vi "top_loop.vi"(0 "Input parameters":T4={"Measurement type"=enum."Debug", "Sensor type"=enum."HPK_8in_256", "Identifier"="test.txt", "Open after execution?"=FALSE, "Plot after execution?"=FALSE, "Display channel"=0, "Voltage Delay (s)"=0.5, "Switch Delay (s)"=0.01, "VISA resource name source"="", "VISA resource name DMM"="", "VISA resource name LCR"="", "Compliance  Level (A)"=10.0, "Voltage Limit (V)"=1000.0, "Data storage location"="", "Scan voltages"="", "Use source as DMM?"=FALSE, "LCR signal frequenzy (Hz)"=10.0, "DMM device"=enum."Keithley2001", "Sampling number"=1, "Use env. sensors on"=enum."Sensirion sht1x/7x", "Switchboard Handle"=0, "Use Switchboard"=FALSE, "LCR signal voltage (V)"=10000.0, "Repeat"=1, "Scan voltages IV"="", "Scan voltages CV"="", "Hex pad numbers?"=FALSE, "Set measurement type"=enum."Debug", "Custom pad scan"="", "IV voltage Delay (s)"=0.5, "CV voltage Delay (s)"=0.5, "Needle measurement?"=FALSE, "Comments"="test.txt", "LCR signal frequenzy (kHz)"=10.0, "Compliance  Level (uA)"=10.0, "Open Correction Array"=array2304x3[6912 elements], "Current set voltage"=0.0, "Last set voltage"=0.0, "Current channel"=0, "Last OpenCorrection index"=-1, "Total curr/vltg every x steps"=10, "Current channel iteration"=0, "No CV corrections"=FALSE, "Mapfile"="", "Corrfile"="", "IV voltage file"=path "", "CV voltage file"=path "", "IV Switch Delay (s)"=0.01, "CV Switch Delay (s)"=0.01, "Invert polarity"=FALSE, "Set debug dirs"=FALSE, "Is n on p"=FALSE} {"CV Switch Delay (s)" format="%#_13g"; "IV Switch Delay (s)" format="%#_13g"; "Last set voltage" format="%#_13g"; "Current set voltage" format="%#_13g"; "CV voltage Delay (s)" format="%#_13g"; "IV voltage Delay (s)" format="%#_13g"; "Voltage Limit (V)" format="%#_13g"; "Voltage Delay (s)" format="%#_13g"; "Switch Delay (s)" format="%#_13g"}, 5 "Dynamic data":T3, 7 "Front_panel_refs":T1, 11 "error in (no error)":errorcluster, 12 "Environmental data":T2) -> (4 "Input parameters out":T4={"Measurement type"=enum."Debug", "Sensor type"=enum."HPK_8in_256", "Identifier"="test.txt", "Open after execution?"=FALSE, "Plot after execution?"=FALSE, "Display channel"=0, "Voltage Delay (s)"=0.5, "Switch Delay (s)"=0.01, "VISA resource name source"="", "VISA resource name DMM"="", "VISA resource name LCR"="", "Compliance  Level (A)"=10.0, "Voltage Limit (V)"=1000.0, "Data storage location"="", "Scan voltages"="", "Use source as DMM?"=FALSE, "LCR signal frequenzy (Hz)"=10.0, "DMM device"=enum."Keithley2001", "Sampling number"=1, "Use env. sensors on"=enum."Sensirion sht1x/7x", "Switchboard Handle"=0, "Use Switchboard"=FALSE, "LCR signal voltage (V)"=10000.0, "Repeat"=1, "Scan voltages IV"="", "Scan voltages CV"="", "Hex pad numbers?"=FALSE, "Set measurement type"=enum."Debug", "Custom pad scan"="", "IV voltage Delay (s)"=0.5, "CV voltage Delay (s)"=0.5, "Needle measurement?"=FALSE, "Comments"="test.txt", "LCR signal frequenzy (kHz)"=10.0, "Compliance  Level (uA)"=10.0, "Open Correction Array"=array2304x3[6912 elements], "Current set voltage"=0.0, "Last set voltage"=0.0, "Current channel"=0, "Last OpenCorrection index"=-1, "Total curr/vltg every x steps"=10, "Current channel iteration"=0, "No CV corrections"=FALSE, "Mapfile"="", "Corrfile"="", "IV voltage file"=path "", "CV voltage file"=path "", "IV Switch Delay (s)"=0.01, "CV Switch Delay (s)"=0.01, "Invert polarity"=FALSE, "Set debug dirs"=FALSE, "Is n on p"=FALSE} {"CV Switch Delay (s)" format="%#_13g"; "IV Switch Delay (s)" format="%#_13g"; "Last set voltage" format="%#_13g"; "Current set voltage" format="%#_13g"; "CV voltage Delay (s)" format="%#_13g"; "IV voltage Delay (s)" format="%#_13g"; "Voltage Limit (V)" format="%#_13g"; "Voltage Delay (s)" format="%#_13g"; "Switch Delay (s)" format="%#_13g"}, 6 "Dynamic data out":T3, 8 "Front_panel_refs out":T1, 15 "error out":errorcluster)   [LabVIEW 2016]
doc: "The main loop function of the HexDAQ."
uses:
  input_params.ctl
  data_dynamic.ctl
  <extravilib>/ChannelInstances/Tag-t'Env_data.ctl'/))Channel.ctl
  data_env.ctl
  refs_front_panel.ctl
  data_live.ctl
  <extravilib>/ChannelInstances/Tag-t'Env_data.ctl'/Read With Abort.vi
  <extravilib>/ChannelInstances/Tag-t'Env_data.ctl'/Endpoint.vi
  <extravilib>/ChannelInstances/Tag-t'Env_data.ctl'.lvlib
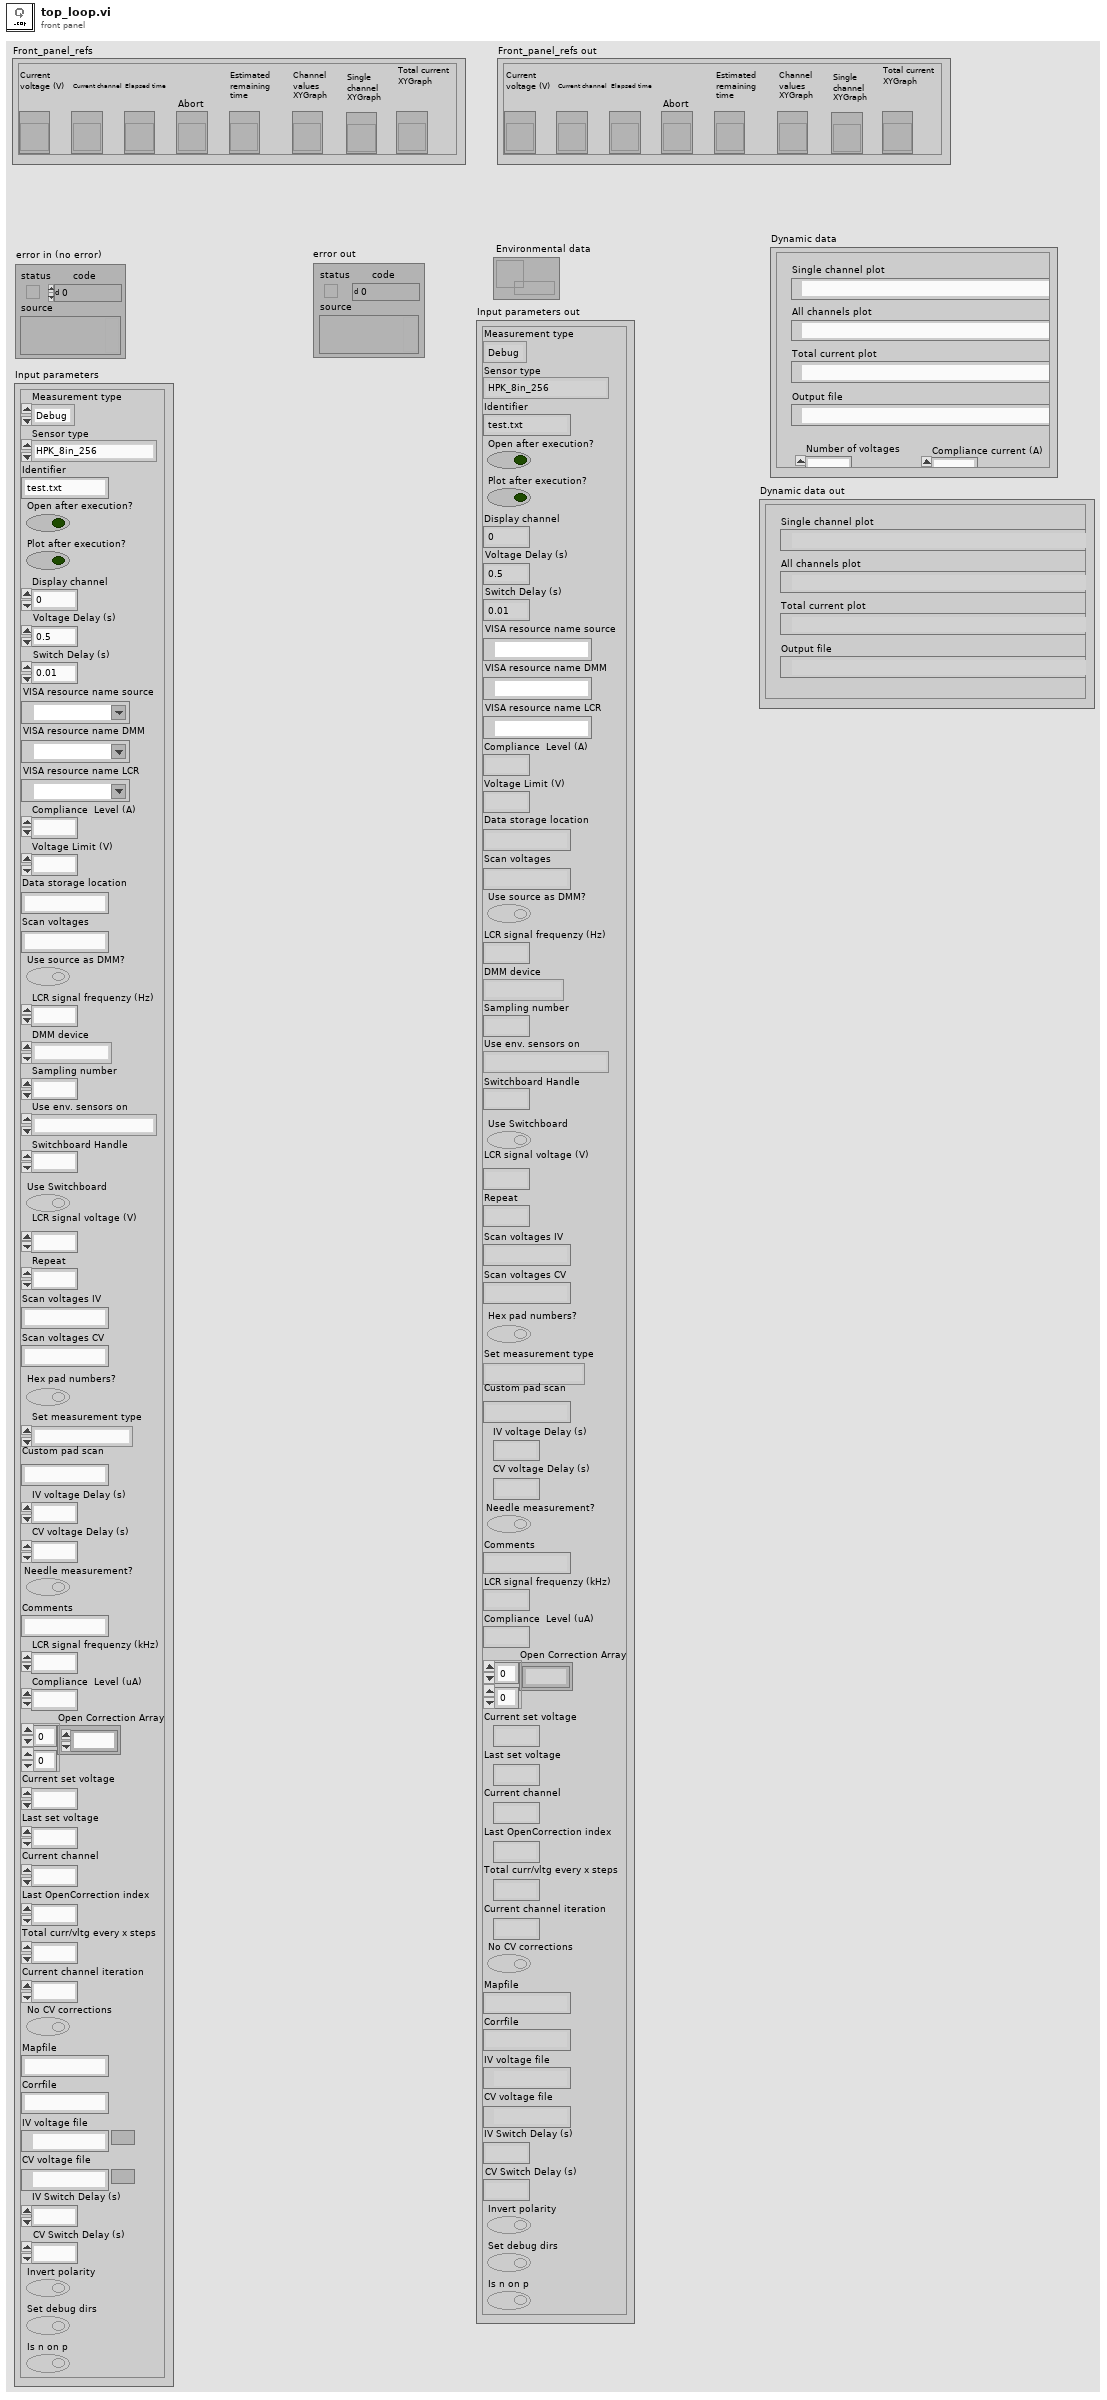
[diagram p1: front panel]
types:
  T1 = typedef "refs_front_panel.ctl" = cluster{"Current voltage (V)":refnum<vi>, "Elapsed time":refnum<vi>, "Current channel":refnum<vi>, "Abort":refnum<vi>, "Estimated remaining time":refnum<vi>, "Channel values XYGraph":refnum<vi>, "Single channel XYGraph":refnum<vi>, "Total current XYGraph":refnum<vi>}
  T2 = typedef "Tag-t'Env_data.ctl'.lvlib/))Channel.ctl" = refnum<queue>
  T3 = typedef "data_dynamic.ctl" = cluster{"Output file":path, "Y-label text":string, "Current set voltage":dbl, "Set voltage column":dbl[], "Pad number column":dbl[], "Data  column":dbl[], "Number of voltages":i32, "Compliance current (A)":dbl, "Geofile":string, "Peak voltage":dbl, "Hex PDF file":string, "Voltage array":dbl[], "Total current column":dbl[], "Timestamp column":dbl[], "Data name":string, "Data unit":string, "2nd data column":dbl[], "2nd data name":string, "2nd data unit":string, "3rd data column":dbl[], "4th data column":dbl[], "3rd data name":string, "3rd data unit":string, "4th data name":string, "4th data unit":string, "Actual voltage column":dbl[], "2nd Y-label text":string, "Single channel plot":path, "Temperature column":dbl[], "Humidity column":dbl[], "Channel switch array":i32[], "1st single plot name":string, "2nd single plot name":string, "All channels plot":path, "HexPlot command":string, "Custom channel array":i32[], "Data  error column":dbl[], "2nd data  error column":dbl[], "3rd data error column":dbl[], "4th data  error column":dbl[], "Total current plot":path, "5th data column":dbl[], "5th data  error column":dbl[], "6th data column":dbl[], "6th data  error column":dbl[], "5th data name":string, "5th data unit":string, "6th data name":string, "6th data unit":string, "HexPlot matrix command":string}
  T4 = typedef "input_params.ctl" = cluster{"Measurement type":enum16{"IV", "CV", "Debug", "Test_contact"}, "Sensor type":enum16{"HPK_6in_135", "HPK_8in_256", "IFX_8in_256", "Diode", "HPK_6in_256", "Full matrix"}, "Identifier":string, "Open after execution?":bool, "Plot after execution?":bool, "Display channel":i32, "Voltage Delay (s)":dbl, "Switch Delay (s)":dbl, "VISA resource name source":refnum<visa-resource-name>, "VISA resource name DMM":refnum<visa-resource-name>, "VISA resource name LCR":refnum<visa-resource-name>, "Compliance  Level (A)":dbl, "Voltage Limit (V)":dbl, "Data storage location":string, "Scan voltages":string, "Use source as DMM?":bool, "LCR signal frequenzy (Hz)":dbl, "DMM device":enum16{"Keithley2001", "Keithley2450", "Keithley2410", "Keithley6487"}, "Sampling number":i32, "Use env. sensors on":enum16{"Sensirion sht1x/7x", "Switch Matrix", "Probecard"}, "Switchboard Handle":u32, "Use Switchboard":bool, "LCR signal voltage (V)":dbl, "Repeat":i32, "Scan voltages IV":string, "Scan voltages CV":string, "Hex pad numbers?":bool, "Set measurement type":enum16{"IV", "CV", "Debug", "Test_contact", "IV+CV"}, "Custom pad scan":string, "IV voltage Delay (s)":dbl, "CV voltage Delay (s)":dbl, "Needle measurement?":bool, "Comments":string, "LCR signal frequenzy (kHz)":dbl, "Compliance  Level (uA)":dbl, "Open Correction Array":dbl[][], "Current set voltage":dbl, "Last set voltage":dbl, "Current channel":i32, "Last OpenCorrection index":i32, "Total curr/vltg every x steps":i32, "Current channel iteration":i32, "No CV corrections":bool, "Mapfile":string, "Corrfile":string, "IV voltage file":path, "CV voltage file":path, "IV Switch Delay (s)":dbl, "CV Switch Delay (s)":dbl, "Invert polarity":bool, "Set debug dirs":bool, "Is n on p":bool}
  T5 = typedef "data_live.ctl" = cluster{"Actual voltage":dbl, "Total current":dbl, "Data":dbl, "Data error":dbl, "2nd data":dbl, "2nd data error":dbl, "3rd data":dbl, "3rd data error":dbl, "4th data":dbl, "4th data error":dbl, "6th data error":dbl, "6th data":dbl, "5th data error":dbl, "5th data":dbl}
  T6 = enum16{"Sensirion sht1x/7x", "Switch Matrix", "Probecard"}
  T7 = typedef "data_env.ctl" = cluster{"Temp. Sensirion":dbl, "Hum. Sensirion":dbl, "Temp. Switch Matrix":dbl, "Hum. Switch Matrix":dbl, "Temp. Probecard":dbl, "Hum. Probecard":dbl}
  T8 = cluster{"XY Graph out":cluster{"Array":dbl[], "Array":dbl[]}[], "XY Graph out":cluster{"Array":dbl[], "Array":dbl[]}[]}
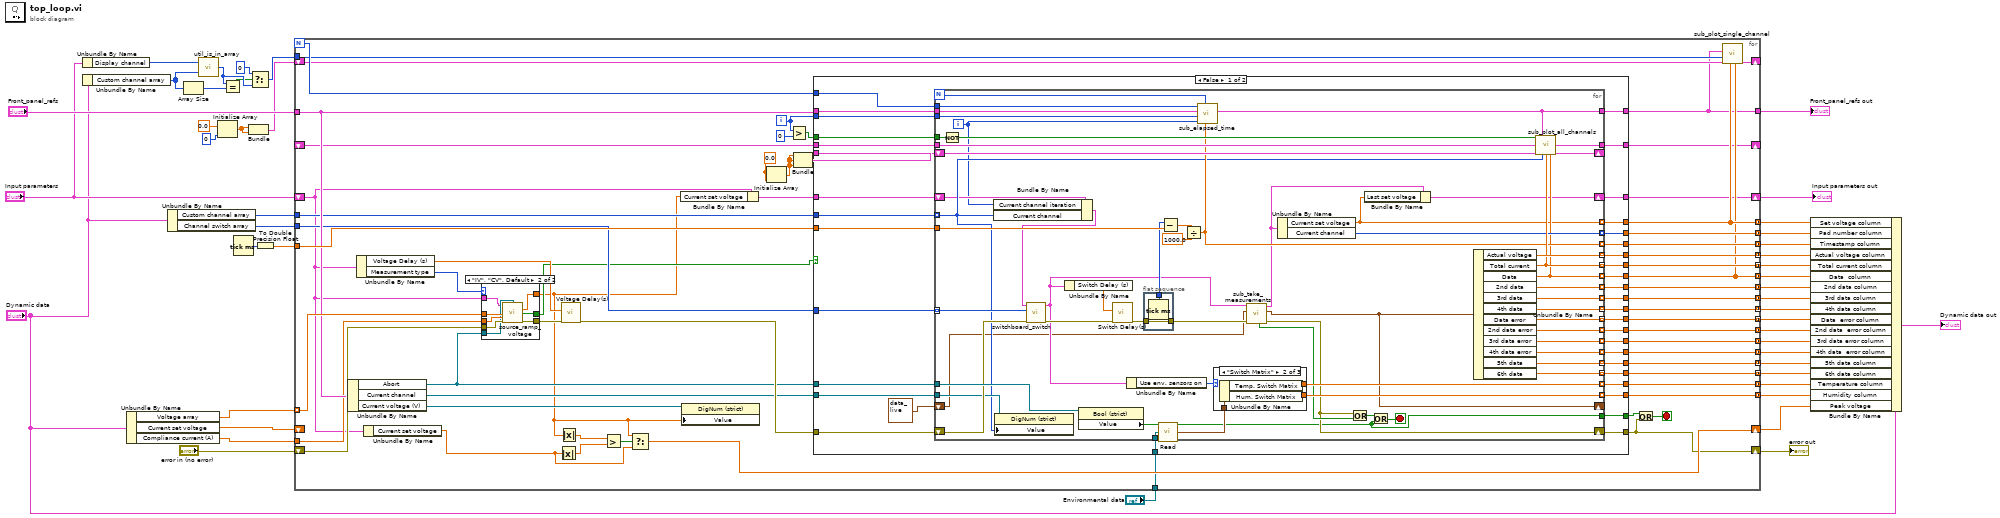
[diagram p0: block diagram]
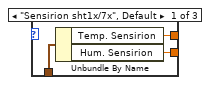
[diagram p2: hidden frame]
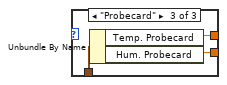
[diagram p3: hidden frame]
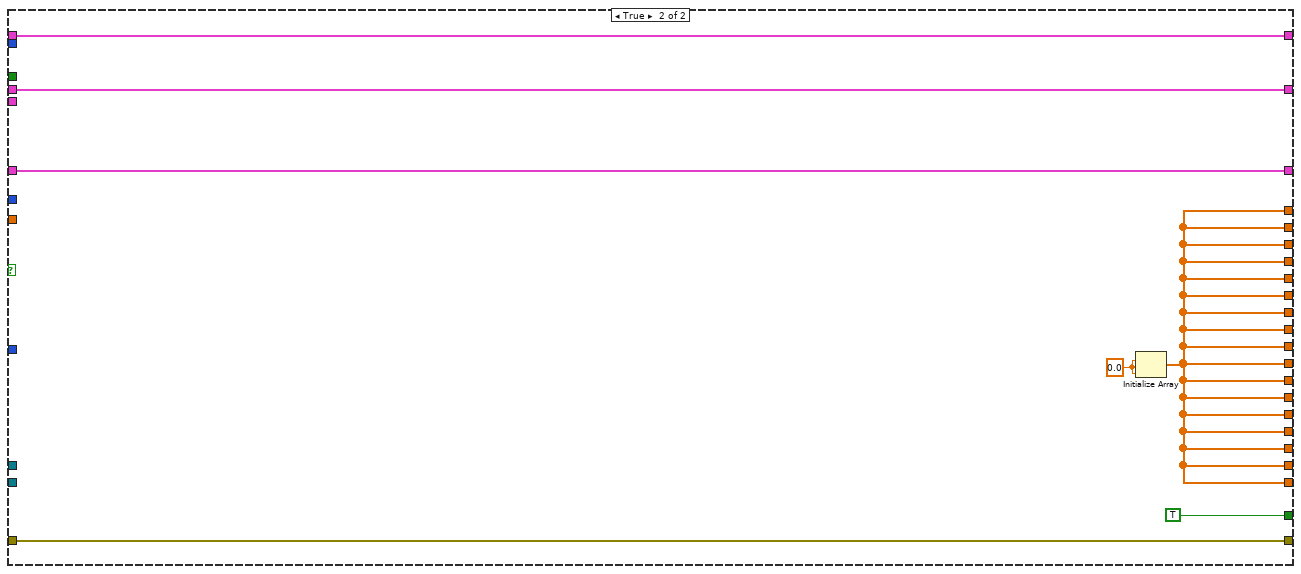
[diagram p4: hidden frame]
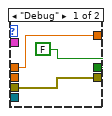
[diagram p5: hidden frame]
diagram:
  n1 = Unbundle By Name("Input parameters") -> ("Display channel"=w23:i32)
  n2 = Unbundle By Name("Dynamic data") -> ("Custom channel array"=w22:i32[])
  n3 = Unbundle By Name("Dynamic data") -> ("Voltage array"=w24:dbl[], "Current set voltage"=w9:dbl, "Compliance current (A)"=w8:dbl)
  n4 = Unbundle By Name("Dynamic data") -> ("Custom channel array"=w15:i32[], "Channel switch array"=w14:i32[])
  n5 = Array Size(array=w22) -> (size(s)=w18:i32)
  n6 = call "util_is_in_array.vi"("Array"=w22, "Numeric"=w23) -> ("Position"=w20:i32)
  n7 = Initialize Array(0.0 ("Secondary Parameter"), 0 ("dimension size")) -> (w11:dbl[])
  n8 = Equal?(x=w20, y=w18) -> (x = y?=w19:bool)
  n9 = Tick Count (ms)() -> (millisecond timer value=w26:u32)
  n10 = Bundle(w11, w11) -> (w10:cluster{dbl[], dbl[]})  [unwired: 1 in]
  n11 = Select(t=0, s=w19, f=w20) -> (s? t:f=w16:i32)
  n12 = To Double Precision Float(number=w26) -> (double precision float=w25:dbl)
  n13 = for {
    N -> [w88]
    tunnel: w24 -> [w96] mode=indexing
    tunnel: [w80] -> w5 mode=concatenating
    tunnel: [w79] -> w45 mode=concatenating
    tunnel: [w102] -> w4 mode=concatenating
    shift-right: [w56] -> w42
    shift-left: "error in (no error)" -> [w101]
    shift-right: [w72] -> w43
    shift-left: "Input parameters" -> [w47]
    tunnel: w25 -> [w92]
    shift-right: [w97] -> w37
    shift-left: w9 -> [_]
    tunnel: [w93] -> w6 mode=concatenating
    tunnel: [w91] -> w7 mode=concatenating
    tunnel: [w90] -> w41 mode=concatenating
    tunnel: [w87] -> w40 mode=concatenating
    tunnel: [w86] -> w39 mode=concatenating
    tunnel: [w85] -> w38 mode=concatenating
    tunnel: [w84] -> w36 mode=concatenating
    tunnel: [w83] -> w35 mode=concatenating
    tunnel: "Environmental data" -> [w82]
    tunnel: [w78] -> w31 mode=concatenating
    tunnel: [w77] -> w30 mode=concatenating
    tunnel: [w76] -> w29 mode=concatenating
    tunnel: [w75] -> w28 mode=concatenating
    tunnel: "Front_panel_refs" -> [w73]
    tunnel: w16 -> [w59]
    tunnel: w8 -> [w68]
    tunnel: w15 -> [w67]
    tunnel: w14 -> [w66]
    shift-right: [w63] -> _
    shift-left: _ -> [w62]
    shift-right: [w60] -> _
    shift-left: w10 -> [w61]
    tunnel: [w54] -> w3 mode=concatenating
    tunnel: [w53] -> w2 mode=concatenating
    tunnel: [w46] -> w1
    i -> [w89]
    stop <- w98 stop-if-true
    w81 = 0.0 ("dimension size")
    n14 = Unbundle By Name(w73) -> ("Abort"=w74:refnum<vi>, "Current channel"=w70:refnum<vi>, "Current voltage (V)"=w71:refnum<vi>)
    n15 = Unbundle By Name(w47) -> ("Voltage Delay (s)"=w69:dbl, "Measurement type"=w95:enum16{"IV", "CV", "Debug", "Test_contact"})
    n16 = Unbundle By Name(w47) -> ("Current set voltage"=w48:dbl)
    n17 = case shown="\"IV\", \"CV\", Default" w95 {
      tunnel: w96 -> [w217 w224]
      tunnel: w101 -> [w218 w225]
      tunnel: [w218 w226] -> w100
      tunnel: w68 -> [_ w223]
      tunnel: [w217 w222] -> w49
      tunnel: w74 -> [_ w221]
      tunnel: [FALSE ("Aborted?") w220] -> w55
      tunnel: w47 -> [_ w219]
      frame "Debug" {
      }
      frame "IV", "CV", Default {
        n18 = call "source_ramp_voltage.vi"("Input parameters"=w219, "Stop"=w221, "Target voltage (V)"=w224, "Compliance Current (A)"=w223, "error in (no error)"=w225) -> ("Current voltage out (V)"=w222:dbl, "Aborted?"=w220:bool, "error out"=w226:errorcluster)  [unwired: 7 in, 1 out]
      }
    }
    n19 = Absolute Value(x=w48) -> (abs(x)=w50:dbl)
    n20 = Absolute Value(x=w49) -> (abs(x)=w51:dbl)
    n21 = call "Voltage Delay(s)"("error in (no error)"=w100, "Delay Time (s)"=w69) -> ("error out"=w94:errorcluster)  [unwired: 9 in]
    n22 = Greater?(x=w51, y=w50) -> (0:w52:bool)
    n23 = Select(t=w49, s=w52, f=w48) -> (s? t:f=w97:dbl)
    n24 = Bundle By Name(cluster=w47, "Current set voltage"=w49) -> (w58:T4)
    n25 = property class="DigNum (strict)"(reference=w71, "Value"=w49) -> ()  [unwired: 1 in, 2 out]
    n26 = Initialize Array(w81, w81) -> (w65:dbl[])
    n27 = Greater?(x=w89, y=0) -> (0:w99:bool)
    n28 = Bundle(w65, w65, w65) -> (w64:cluster{dbl[], dbl[], dbl[]})  [unwired: 1 in]
    n29 = case shown="False" w55 {
      tunnel: [w140 w210] -> w102
      tunnel: w99 -> [w139 _]
      tunnel: w94 -> [w138 w213]
      tunnel: [w137 w210] -> w93
      tunnel: w92 -> [w136 _]
      tunnel: [w135 w210] -> w91
      tunnel: [w134 w210] -> w90
      tunnel: w89 -> [w133 _]
      tunnel: w88 -> [w132 _]
      tunnel: [w131 w210] -> w87
      tunnel: [w130 w210] -> w86
      tunnel: [w129 w210] -> w85
      tunnel: [w128 w210] -> w84
      tunnel: [w127 w210] -> w83
      tunnel: w82 -> [w126 _]
      tunnel: [w125 w210] -> w80
      tunnel: [w124 w210] -> w79
      tunnel: [w123 w210] -> w78
      tunnel: [w122 w210] -> w77
      tunnel: [w121 w210] -> w76
      tunnel: [w120 w210] -> w75
      tunnel: w74 -> [w119 _]
      tunnel: w73 -> [w118 w209]
      tunnel: [w117 w215] -> w72
      tunnel: w70 -> [w116 _]
      tunnel: w67 -> [w115 _]
      tunnel: w66 -> [w114 _]
      tunnel: w64 -> [w113 _]
      tunnel: [w112 w214] -> w63
      tunnel: w62 -> [w111 w214]
      tunnel: w58 -> [w110 w215]
      tunnel: [w109 TRUE ("Value")] -> w57
      tunnel: [w108 w213] -> w56
      tunnel: [w107 w210] -> w53
      tunnel: [w106 w210] -> w54
      tunnel: [w104 w209] -> w46
      frame False {
        n30 = for {
          N -> [w161]
          tunnel: w114 -> [w182] mode=indexing
          tunnel: [w158] -> w140 mode=indexing
          tunnel: [w155] -> w124 mode=indexing
          tunnel: [w145] -> w125 mode=indexing
          shift-right: [w153] -> w108
          shift-left: w138 -> [w184]
          tunnel: w139 -> [w176]
          tunnel: [w151] -> w109
          tunnel: w119 -> [w197]
          tunnel: [w164] -> w137 mode=indexing
          tunnel: w136 -> [w196]
          tunnel: [w162] -> w135 mode=indexing
          tunnel: [w175] -> w134 mode=indexing
          tunnel: w133 -> [w169]
          tunnel: w132 -> [w160]
          tunnel: [w191] -> w131 mode=indexing
          tunnel: [w190] -> w130 mode=indexing
          tunnel: [w189] -> w129 mode=indexing
          tunnel: [w187] -> w128 mode=indexing
          tunnel: [w186] -> w127 mode=indexing
          tunnel: w126 -> [w185]
          tunnel: w115 -> [w159] mode=indexing
          tunnel: [w180] -> w123 mode=indexing
          tunnel: [w179] -> w122 mode=indexing
          tunnel: [w178] -> w121 mode=indexing
          tunnel: [w177] -> w120 mode=indexing
          tunnel: w116 -> [w172]
          tunnel: w118 -> [w168]
          shift-right: [w167] -> _
          shift-left: w113 -> [w163]
          tunnel: [w165] -> w112
          tunnel: w111 -> [w166]
          shift-right: [w147] -> w117
          shift-left: w110 -> [w157]
          tunnel: [w149] -> w107 mode=indexing
          tunnel: [w148] -> w106 mode=indexing
          shift-right: [w144] -> _
          shift-left: T5 {"Actual voltage"=0.0, "Total current"=0.0, "Data"=0.0, "Data error"=0.0, "2nd data"=0.0, "2nd data error"=0.0, "3rd data"=0.0, "3rd data error"=0.0, "4th data"=0.0, "4th data error"=0.0, "6th data error"=0.0, "6th data"=0.0, "5th data error"=0.0, "5th data"=0.0} ("Live data out") -> [w143]
          tunnel: [w141] -> w104
          i -> [w142]
          stop <- w150 stop-if-true
          n31 = Not(x=w176) -> (.not. x?=w174:bool)
          n32 = Bundle By Name(cluster=w157, "Current channel iteration"=w142, "Current channel"=w159) -> (w156:T4)
          n33 = property on="Property Node" class="DigNum (strict)"(reference=w172, "Value"=w159) -> ()  [unwired: 1 in, 2 out]
          n34 = call "switchboard_switch.vi"("error in"=w184, "Channel"=w182, "Input parameters in"=w156) -> ("error out"=w183:errorcluster, "Input parameters out"=w170:T4)  [unwired: 7 in]
          n35 = Unbundle By Name(w170) -> ("Switch Delay (s)"=w173:dbl)
          n36 = property class="Bool (strict)"(reference=w197) -> ("Value"=w151:bool)  [unwired: 1 in, 2 out]
          n37 = call "Switch Delay(s)"("error in (no error)"=w183, "Delay Time (s)"=w173) -> ("error out"=w193:errorcluster)  [unwired: 9 in]
          n38 = Unbundle By Name(w170) -> ("Use env. sensors on"=w181:T6)
          n39 = flat-sequence {
            tunnel: [w208] -> w194
            tunnel: w193 -> [w207]
            tunnel: [w207] -> w192
            frame #0 {
              n40 = Tick Count (ms)() -> (millisecond timer value=w208:u32)
            }
          }
          n41 = call <extravilib>:"Read.vi"("channel"=w185) -> ("element"=w188:T7)  [unwired: 1 in, 1 out]
          n42 = Subtract(x=w194, y=w196) -> (x-y=w171:dbl)
          n43 = Divide(x=w171, y=1000.0) -> (x/y=w162:dbl)
          n44 = call "sub_elapsed_time.vi"("Elapsed time (s)"=w162, "Inner N"=w161, "Inner i"=w142, "Outer i"=w169, "Front_panel_refs"=w168, "Outer N"=w160) -> ("Front_panel_refs out"=w141:T1)  [unwired: 5 in]
          n45 = case shown="\"Switch Matrix\"" w181 {
            tunnel: w188 -> [w200 w203 w206]
            tunnel: [w199 w201 w204] -> w187
            tunnel: [w198 w202 w205] -> w186
            frame "Sensirion sht1x/7x", Default {
              n46 = Unbundle By Name(w200) -> ("Temp. Sensirion"=w199:dbl, "Hum. Sensirion"=w198:dbl)
            }
            frame "Switch Matrix" {
              n47 = Unbundle By Name(w203) -> ("Temp. Switch Matrix"=w201:dbl, "Hum. Switch Matrix"=w202:dbl)
            }
            frame "Probecard" {
              n48 = Unbundle By Name(w206) -> ("Temp. Probecard"=w204:dbl, "Hum. Probecard"=w205:dbl)
            }
          }
          n49 = call "sub_take_measurements.vi"("error in (no error)"=w192, "Live data in"=w143, "Input parameters"=w170) -> ("error out"=w153:errorcluster, "Live data out"=w144:T5, "Input parameters out"=w146:T4, "Compliance reached?"=w154:bool)  [unwired: 5 in]
          n50 = Unbundle By Name(w146) -> ("Current set voltage"=w145:dbl, "Current channel"=w158:i32)
          n51 = Or(x=w153, y=w154) -> (x .or. y?=w152:bool)
          n52 = Bundle By Name(cluster=w146, "Last set voltage"=w145) -> (w147:T4)
          n53 = Or(x=w152, y=w151) -> (x .or. y?=w150:bool)
          n54 = Unbundle By Name(w144) -> ("Actual voltage"=w189:dbl, "Total current"=w164:dbl, "Data"=w155:dbl, "2nd data"=w175:dbl, "3rd data"=w191:dbl, "4th data"=w190:dbl, "Data error"=w180:dbl, "2nd data error"=w179:dbl, "3rd data error"=w178:dbl, "4th data error"=w177:dbl, "5th data"=w149:dbl, "6th data"=w148:dbl)
          n55 = call "sub_plot_all_channels.vi"("Is first?"=w174, "Front_panel_refs"=w141, "Plot cluster"=w166, "Cluster"=w163, "Custom channel"=w159, "Total current"=w164, "Data"=w155) -> ("Plot cluster out"=w165:T8, "Cluster out"=w167:cluster{dbl[], dbl[], dbl[]})  [unwired: 7 in]
        }
      }
      frame True {
        w211 = 0.0 ("dimension size")
        n56 = Initialize Array(w211, w211) -> (w210:dbl[])
      }
    }
    n57 = Or(x=w57, y=w56) -> (x .or. y?=w98:bool)
    n58 = call "sub_plot_single_channel.vi"("Data column"=w79, "Set voltage column"=w80, "Cluster"=w61, "Channel"=w59, "Front_panel_refs"=w46) -> ("Cluster out"=w60:cluster{dbl[], dbl[]})  [unwired: 6 in]
  }
  "error out" <- w42
  "Input parameters out" <- w43
  "Front_panel_refs out" <- w1
  n59 = Bundle By Name(cluster="Dynamic data", "Set voltage column"=w5, "Pad number column"=w4, "Timestamp column"=w7, "Actual voltage column"=w38, "Total current column"=w6, "Data  column"=w45, "2nd data column"=w41, "3rd data column"=w40, "4th data column"=w39, "Data  error column"=w31, "2nd data  error column"=w30, "3rd data error column"=w29, "4th data  error column"=w28, "5th data column"=w2, "6th data column"=w3, "Temperature column"=w36, "Humidity column"=w35, "Peak voltage"=w37) -> (→"Dynamic data out":T3)
